vi "ParseValue.vi"(5 "payload":string, 6 "error in":errorcluster) -> (0 "error out":errorcluster, 4 "value":string)   [LabVIEW 2014, in "Raspberry Pi Compatible Compiler for LabVIEW.lvlib" / "RasPiDownloader.lvlib"]
uses:
  RasPiDownloader.lvlib
  MessageWithValueTD.ctl
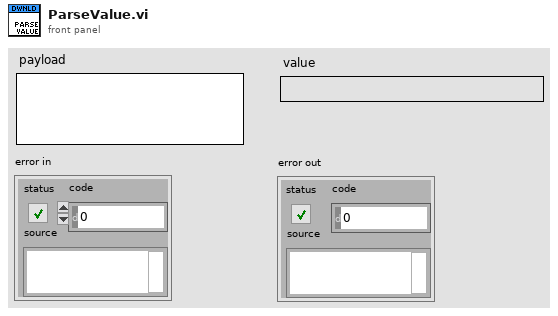
[diagram p1: front panel]
types:
  T1 = typedef "Raspberry Pi Compatible Compiler for LabVIEW.lvlib/RasPiDownloader.lvlib/MessageWithValueTD.ctl" = cluster{"cmd":string, "value":string}
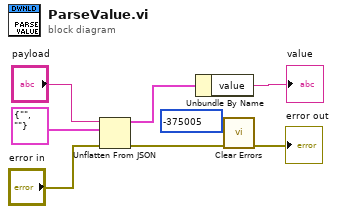
[diagram p0: block diagram]
diagram:
  n1 = Unflatten From JSON(JSON string="payload", type and defaults=T1 {"cmd"="", "value"=""} ("message"), error in (no error)="error in") -> (value=w5:T1, error out=w3:errorcluster)  [unwired: 4 in]
  n2 = Unbundle By Name(w5) -> ("value"=→"value":string)
  n3 = call <vilib>:"Clear Errors.vi"("error in (no error)"=w3, "specific error code to clear (0: all)"=-375005) -> ("error out"=→"error out":errorcluster)  [unwired: 4 in, 1 out]
